vi "Set_Sweep_Wavelength.vi"(8 "error in (no error)":errorcluster, 9 "Stop wavelength":dbl, 10 "Start wavelength":dbl, 11 ".NET Reference in":refnum<k24>) -> (0 "error out":errorcluster, 3 ".NET Reference out":refnum<k24>)   [LabVIEW 2017]
uses:
  C:/Users/Ssantec_Test/Documents/Instrument_DLL_Sample_Labview_20220902_Ver1.2.2/DLL/x86/InstrumentDLL.dll
  DLL/x86/InstrumentDLL.dll
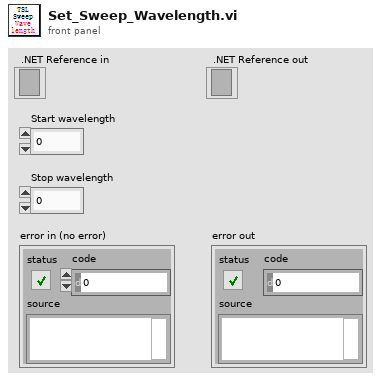
[diagram p1: front panel]
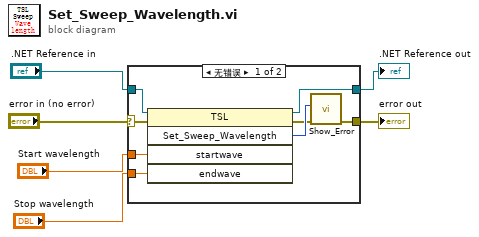
[diagram p0: block diagram]
diagram:
  n1 = case shown="无错误" "error in (no error)" {
    selector: "error in (no error)" -> [w7 w16]
    tunnel: "Stop wavelength" -> [w14 _]
    tunnel: "Start wavelength" -> [w13 _]
    tunnel: [w8 w16] -> w4
    tunnel: [w12 w15] -> w3
    tunnel: ".NET Reference in" -> [w11 w15]
    frame No Error {
      n2 = invoke on="调用节点" class="TSL" method="Set_Sweep_Wavelength"(reference=w11, error in=w7, "startwave"=w13, "endwave"=w14) -> (reference out=w12:refnum<k24>, error out=w9:errorcluster, "Set_Sweep_Wavelength"=w10:i32)  [unwired: 1 in, 2 out]
      n3 = call "Show_Error.vi"("error in (no error)"=w9, "Error"=w10) -> ("error out"=w8:errorcluster)  [unwired: 9 in]
    }
    frame Error {
    }
  }
  "error out" <- w4
  ".NET Reference out" <- w3
